vi "WholeRunProcess-Tiepie-2018-04-26.vi"() -> ()   [LabVIEW 2013]
panel:
  in  "ShutDownSystem":bool
  out "XY Graph":cluster{dbl[], "Intensity_Total":sgl[]}(graph)
  out "Card-OK":bool
  in  "Start":bool
  in  "ShotsPerPoint":u16=100
  in  "Record Length/Samples":u64=50000
  in  "Sample Frequency/Hz":i32=200000000
  in  "TiepieID":i32=33474
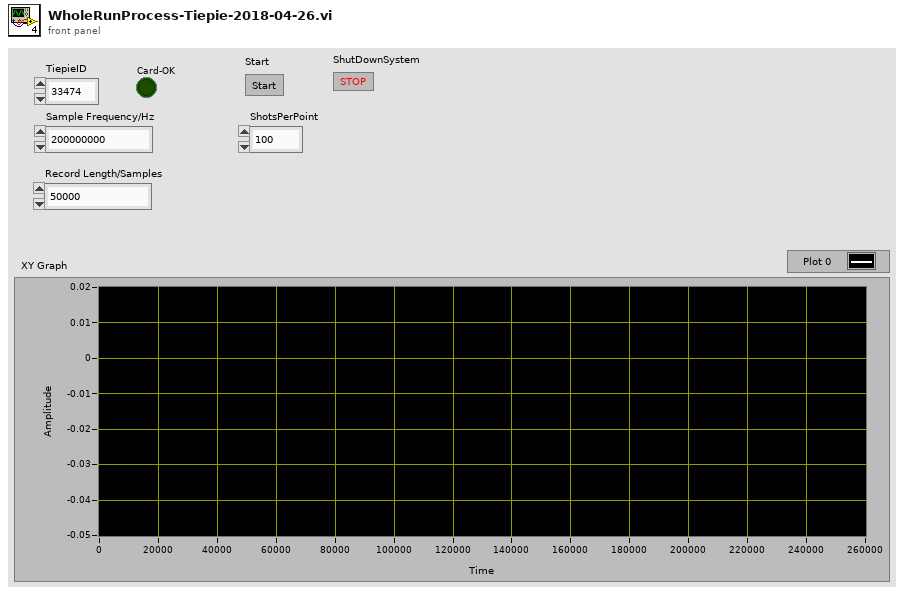
[diagram p1: front panel]
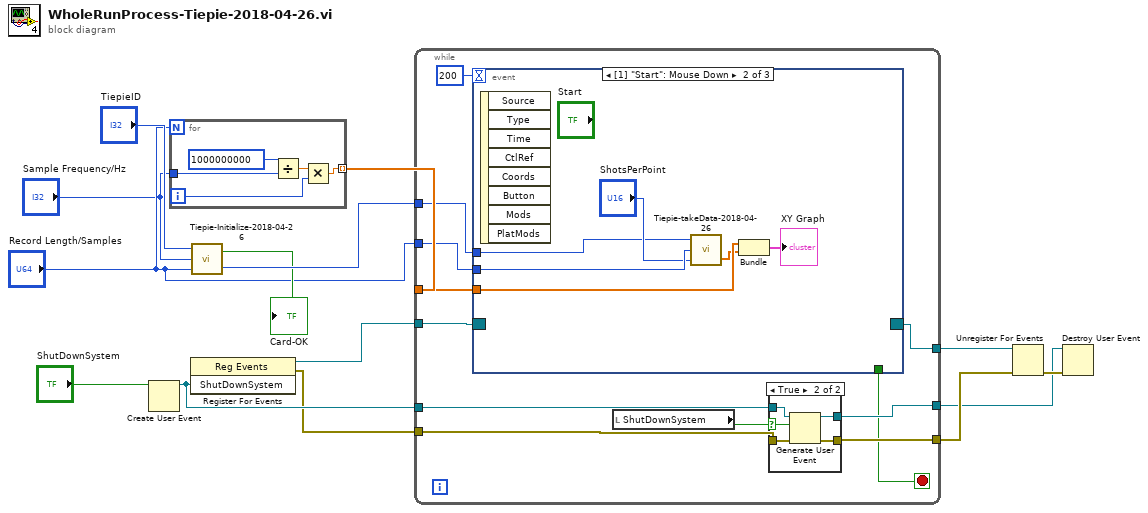
[diagram p0: block diagram]
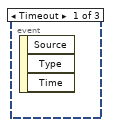
[diagram p3: hidden frame]
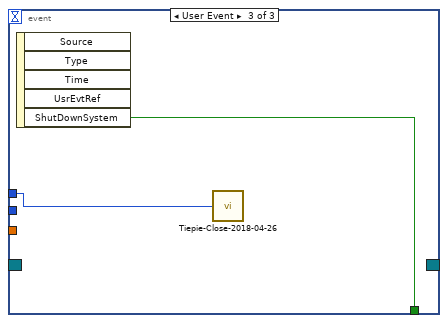
[diagram p4: hidden frame]
diagram:
  n1 = Create User Event(user event datatype="ShutDownSystem") -> (user event=w6:refnum<user-event>)  [unwired: 1 in, 1 out]
  n2 = for {
    N: "Record Length/Samples" -> [_]
    tunnel: "Sample Frequency/Hz" -> [w18]
    tunnel: [w15] -> w9 mode=indexing
    i -> [w16]
    n3 = Divide(x=1000000000, y=w18) -> (x/y=w17:dbl)
    n4 = Multiply(x=w17, y=w16) -> (x*y=w15:dbl)
  }
  n5 = register-events(w6) -> (reference out=w7:refnum<event-registration>, error out=w5:errorcluster)  [unwired: 2 in]
  n6 = call "Tiepie-Initialize-2018-04-26.vi"("Record Length/Samples"="Record Length/Samples", "Sample Frequency/Hz"="Sample Frequency/Hz", "TiepieID"="TiepieID") -> ("TpDeviceHandle_t"=w13:u32, "Card-OK"=→"Card-OK":bool)
  n7 = while {
    tunnel: w13 -> [w31]
    tunnel: "Record Length/Samples" -> [w30]
    tunnel: w9 -> [w29]
    tunnel: w7 -> [w28]
    tunnel: w6 -> [w26]
    tunnel: w5 -> [w25]
    tunnel: [w24] -> w4
    tunnel: [w23] -> w2
    tunnel: [w22] -> w1
    stop <- w20 stop-if-true
    n8 = event shown="[1] \"Start\": Mouse Down" {
      selector: w28 -> [_ _ _]
      dyn-events: [_ _ _] -> w23
      timeout: 200 -> [_ _ _]
      tunnel: w31 -> [_ w39 w45]
      tunnel: w30 -> [_ w41 _]
      tunnel: w29 -> [_ w44 _]
      tunnel: [_ _ w46] -> w20
      event Timeout {
        n9 = event-data() -> ()  [unwired: 1 in, 3 out]
      }
      event "Start": Mouse Down {
        n10 = event-data() -> ()  [unwired: 1 in, 8 out]
        n11 = call "Tiepie-takeData-2018-04-26.vi"("ShotsPerPoint"="ShotsPerPoint", "Record Length/Samples"=w41, "TpDeviceHandle_t"=w39) -> ("Intensity_Total"=w42:sgl[])  [unwired: 1 out]
        n12 = Bundle(w44, "Intensity_Total"=w42) -> (→"XY Graph":cluster{dbl[], "Intensity_Total":sgl[]})  [unwired: 1 in]
      }
      event User Event {
        n13 = event-data() -> ("ShutDownSystem"=w46:bool)  [unwired: 1 in, 4 out]
        n14 = call "Tiepie-Close-2018-04-26.vi"("TpDeviceHandle_t"=w45) -> ()
      }
    }
    n15 = local read "ShutDownSystem"() -> (w27:bool)
    n16 = case shown="True" w27 {
      selector: w27 -> [_ w37]
      tunnel: w26 -> [w33 w38]
      tunnel: w25 -> [w32 w36]
      tunnel: [w32 w35] -> w24
      tunnel: [w33 w34] -> w22
      frame False {
      }
      frame True {
        n17 = Generate User Event(user event=w38, event data cluster=w37, error in=w36) -> (user event out=w34:refnum<user-event>, error out=w35:errorcluster)  [unwired: 1 in]
      }
    }
  }
  n18 = Unregister For Events(event registration refnum=w2, error in=w4) -> (error out=w3:errorcluster)
  n19 = Destroy User Event(user event=w1, error in=w3) -> ()  [unwired: 1 out]
